vi "Dashboard Main.vi"() -> ()   [LabVIEW 2011]
uses:
  <vilib>/Rock Robotics/WPI/DriverStation/DriverStationLCD/WPI_DriverStationLCDLCDLine.ctl
  DStoPCPacketTypeDef.ctl
  <vilib>/Rock Robotics/WPI/DriverStation/WPI_DriverStationDigitalData.ctl
panel:
  out "SPEED":dbl(knob) scale=0.1..100.0
  out "8 -- Battery":sgl(graph)
  out "Analog Input":sgl[](array[slide]) scale=0.0..5.0
  in  "Viewer":enum32{"Camera Image", "Kinect Skeleton"}(tab)
  in  "Video Enable":bool=TRUE
  out "Camera Image":T1(plugin-control)
  out "Buttons 1":cluster{"1":bool, "2":bool, "3":bool}
  out "Kinect 1":cluster{"X":dbl, "Y":dbl, "Z":dbl} {"X" scale=1.0..-1.0; "Y" scale=1.0..-1.0; "Z" scale=1.0..-1.0}
  out "Buttons 2":cluster{"1":bool, "2":bool, "3":bool}
  out "Kinect 2":cluster{"X":dbl, "Y":dbl, "Z":dbl} {"X" scale=1.0..-1.0; "Y" scale=1.0..-1.0; "Z" scale=1.0..-1.0}
  out "Version":string
  out "Skeleton Picture":picture
  out "Players":i8
  out "Dashboard Datatype Warning":string="Warning: The Dashboard Datatype used by the robot project and this dashboard do not match.\nSee diagram for more details."
  out "Robot IP Address":string
  out "Image Error Message":string="Timeout in Camera Communications"
  out "Solenoid Output":bool[](array[boolean])
  out "PWM":cluster{u8, u8}[](array[slide])=[{0, 157}, {0, 157}, {0, 157}, {0, 157}, {0, 157}, {0, 157}, {0, 157}, {0, 157}, {0, 157}, {0, 169}] scale=1.0..255.0
  out "GPIO Output Enable":bool[](array[boolean])
  out "GPIO State":bool[](array[boolean])
  out "Relay":cluster{"Forward":bool[], "Reverse":bool[]}
  # "Analog #1"
  # "1"
  # "7"
  # "Communications"
  # "Solenoid #1"
  # "1"
  # "8"
  # "Digital #1"
  # "1"
  # "10"
  # "1"
  # "14"
  # "1"
  # "8"
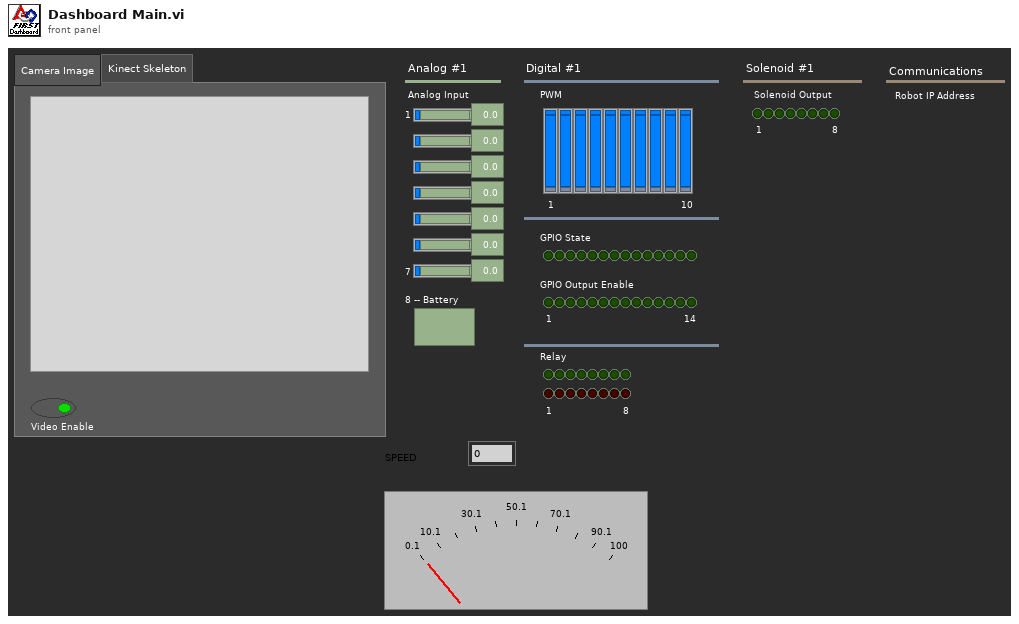
[diagram p1: front panel]
types:
  T1 = typedef "IMAQ Image.ctl" = refnum<image>
  T2 = typedef "DStoPCPacketTypeDef.ctl" = cluster{"Packet Index":u16, "Digital Inputs":u8, "Digital Out":u8, "Battery":u16, "Status":u8, "Error":u8, "Team ID":u16, "VersionMonth1":u8, "VersionMonth2":u8, "VersionDay1":u8, "VersionDay2":u8, "VersionYear1":u8, "VersionYear2":u8, "Revision1":u8, "Revision2":u8, "UnusedBuffer":u32, "UnusedBuffer 2":u16, "Reply Packet #":u16, "SPEED":dbl}
  T3 = cluster{"AnalogModule[0]":cluster{"Channel[3]":sgl}, "AnalogModule[1]":cluster{"Channel[1]":sgl}, "Cluster":T2}
  T4 = typedef "WPI_DriverStationDigitalData.ctl" = cluster{"Relay Fwd":u8, "Relay Rev":u8, "GPIO":u16, "GPIO_OE":u16, "PWM":cluster{"PWM[0]":u8, "PWM[1]":u8, "PWM[2]":u8, "PWM[3]":u8, "PWM[4]":u8, "PWM[5]":u8, "PWM[6]":u8, "PWM[7]":u8, "PWM[8]":u8, "PWM[9]":u8}}
  T5 = cluster{cluster{"AnalogModule[0]":cluster{"Channel[0]":sgl, "Channel[1]":sgl, "Channel[2]":sgl, "Channel[3]":sgl, "Channel[4]":sgl, "Channel[5]":sgl, "Channel[6]":sgl, "Channel[7]":sgl}, "AnalogModule[1]":cluster{"Channel[0]":sgl, "Channel[1]":sgl, "Channel[2]":sgl, "Channel[3]":sgl, "Channel[4]":sgl, "Channel[5]":sgl, "Channel[6]":sgl, "Channel[7]":sgl}}, cluster{"DigitalModule[0]":T4}, "Solenoid":u8, "DigitalModule[1]":T4}
  T6 = typedef "Image Type" = u32
  T7 = cluster{"Competition mode":bool, "Robot Link":bool, "Autonomous":bool, "Enabled":bool, "E-Stop":bool}
  T8 = cluster{"AnalogModule[0]":cluster{"Channel[0]":sgl, "Channel[1]":sgl, "Channel[2]":sgl, "Channel[3]":sgl, "Channel[4]":sgl, "Channel[5]":sgl, "Channel[6]":sgl, "Channel[7]":sgl}, "AnalogModule[1]":cluster{"Channel[0]":sgl, "Channel[1]":sgl, "Channel[2]":sgl, "Channel[3]":sgl, "Channel[4]":sgl, "Channel[5]":sgl, "Channel[6]":sgl, "Channel[7]":sgl}}
  T9 = cluster{"Channel[0]":sgl, "Channel[1]":sgl, "Channel[2]":sgl, "Channel[3]":sgl, "Channel[4]":sgl, "Channel[5]":sgl, "Channel[6]":sgl, "Channel[7]":sgl}[]
  T10 = cluster{"Channel[0]":sgl, "Channel[1]":sgl, "Channel[2]":sgl, "Channel[3]":sgl, "Channel[4]":sgl, "Channel[5]":sgl, "Channel[6]":sgl, "Channel[7]":sgl}
  T11 = typedef "LVRectTypeDef.ctl" = cluster{"left":i16, "top":i16, "right":i16, "bottom":i16}
  T12 = typedef "SkeletonTrackState.ctl" = enum32{"NotTracked", "PositionOnly", "Tracked"}
  T13 = cluster{"TrackingState":u8[], "Position":cluster{"x":sgl, "y":sgl, "z":sgl}, cluster{"x":sgl, "y":sgl, "z":sgl, sgl}[], "TrackState":T12}
  T14 = cluster{cluster{"ScaledToPercentRange":dbl, "ScaledToPercentRange":dbl, "ScaledToPercentRange":dbl}, cluster{bool, bool, bool}}[]
  T15 = typedef "LVBoundsTypeDef.ctl" = cluster{"Width":u32, "Height":u32}
  T16 = cluster{cluster{"ScaledToPercentRange":dbl, "ScaledToPercentRange":dbl, "ScaledToPercentRange":dbl}, cluster{bool, bool, bool}}
  T17 = cluster{"ScaledToPercentRange":dbl, "ScaledToPercentRange":dbl, "ScaledToPercentRange":dbl}
  T18 = typedef "WPI_DriverStationLCDLCDLine.ctl" = enum16{"Main - Line 1", "User - Line 2", "User - Line 3", "User - Line 4", "User - Line 5", "User - Line 6"}
  T19 = typedef "WPI_EncoderDevRef.ctl" = cluster{"DevStatus":errorcluster, "EncoderIndex":T20, "CounterIndex":T21, "DistancePerCount":dbl, "Decoding Type":T22}
  T20 = typedef "FPGA_EncoderIdx.ctl" = enum8{"Enc 0", "Enc 1", "Enc 2", "Enc 3", "Invalid"}
  T21 = typedef "FPGA_CounterCtrSystemIndex.ctl" = enum8{"Ctr 0", "Ctr 1", "Ctr 2", "Ctr 3", "Ctr 4", "Ctr 5", "Ctr 6", "Ctr 7", "Invalid"}
  T22 = typedef "WPI_EncoderType.ctl" = enum16{"1x", "2x", "4x"}
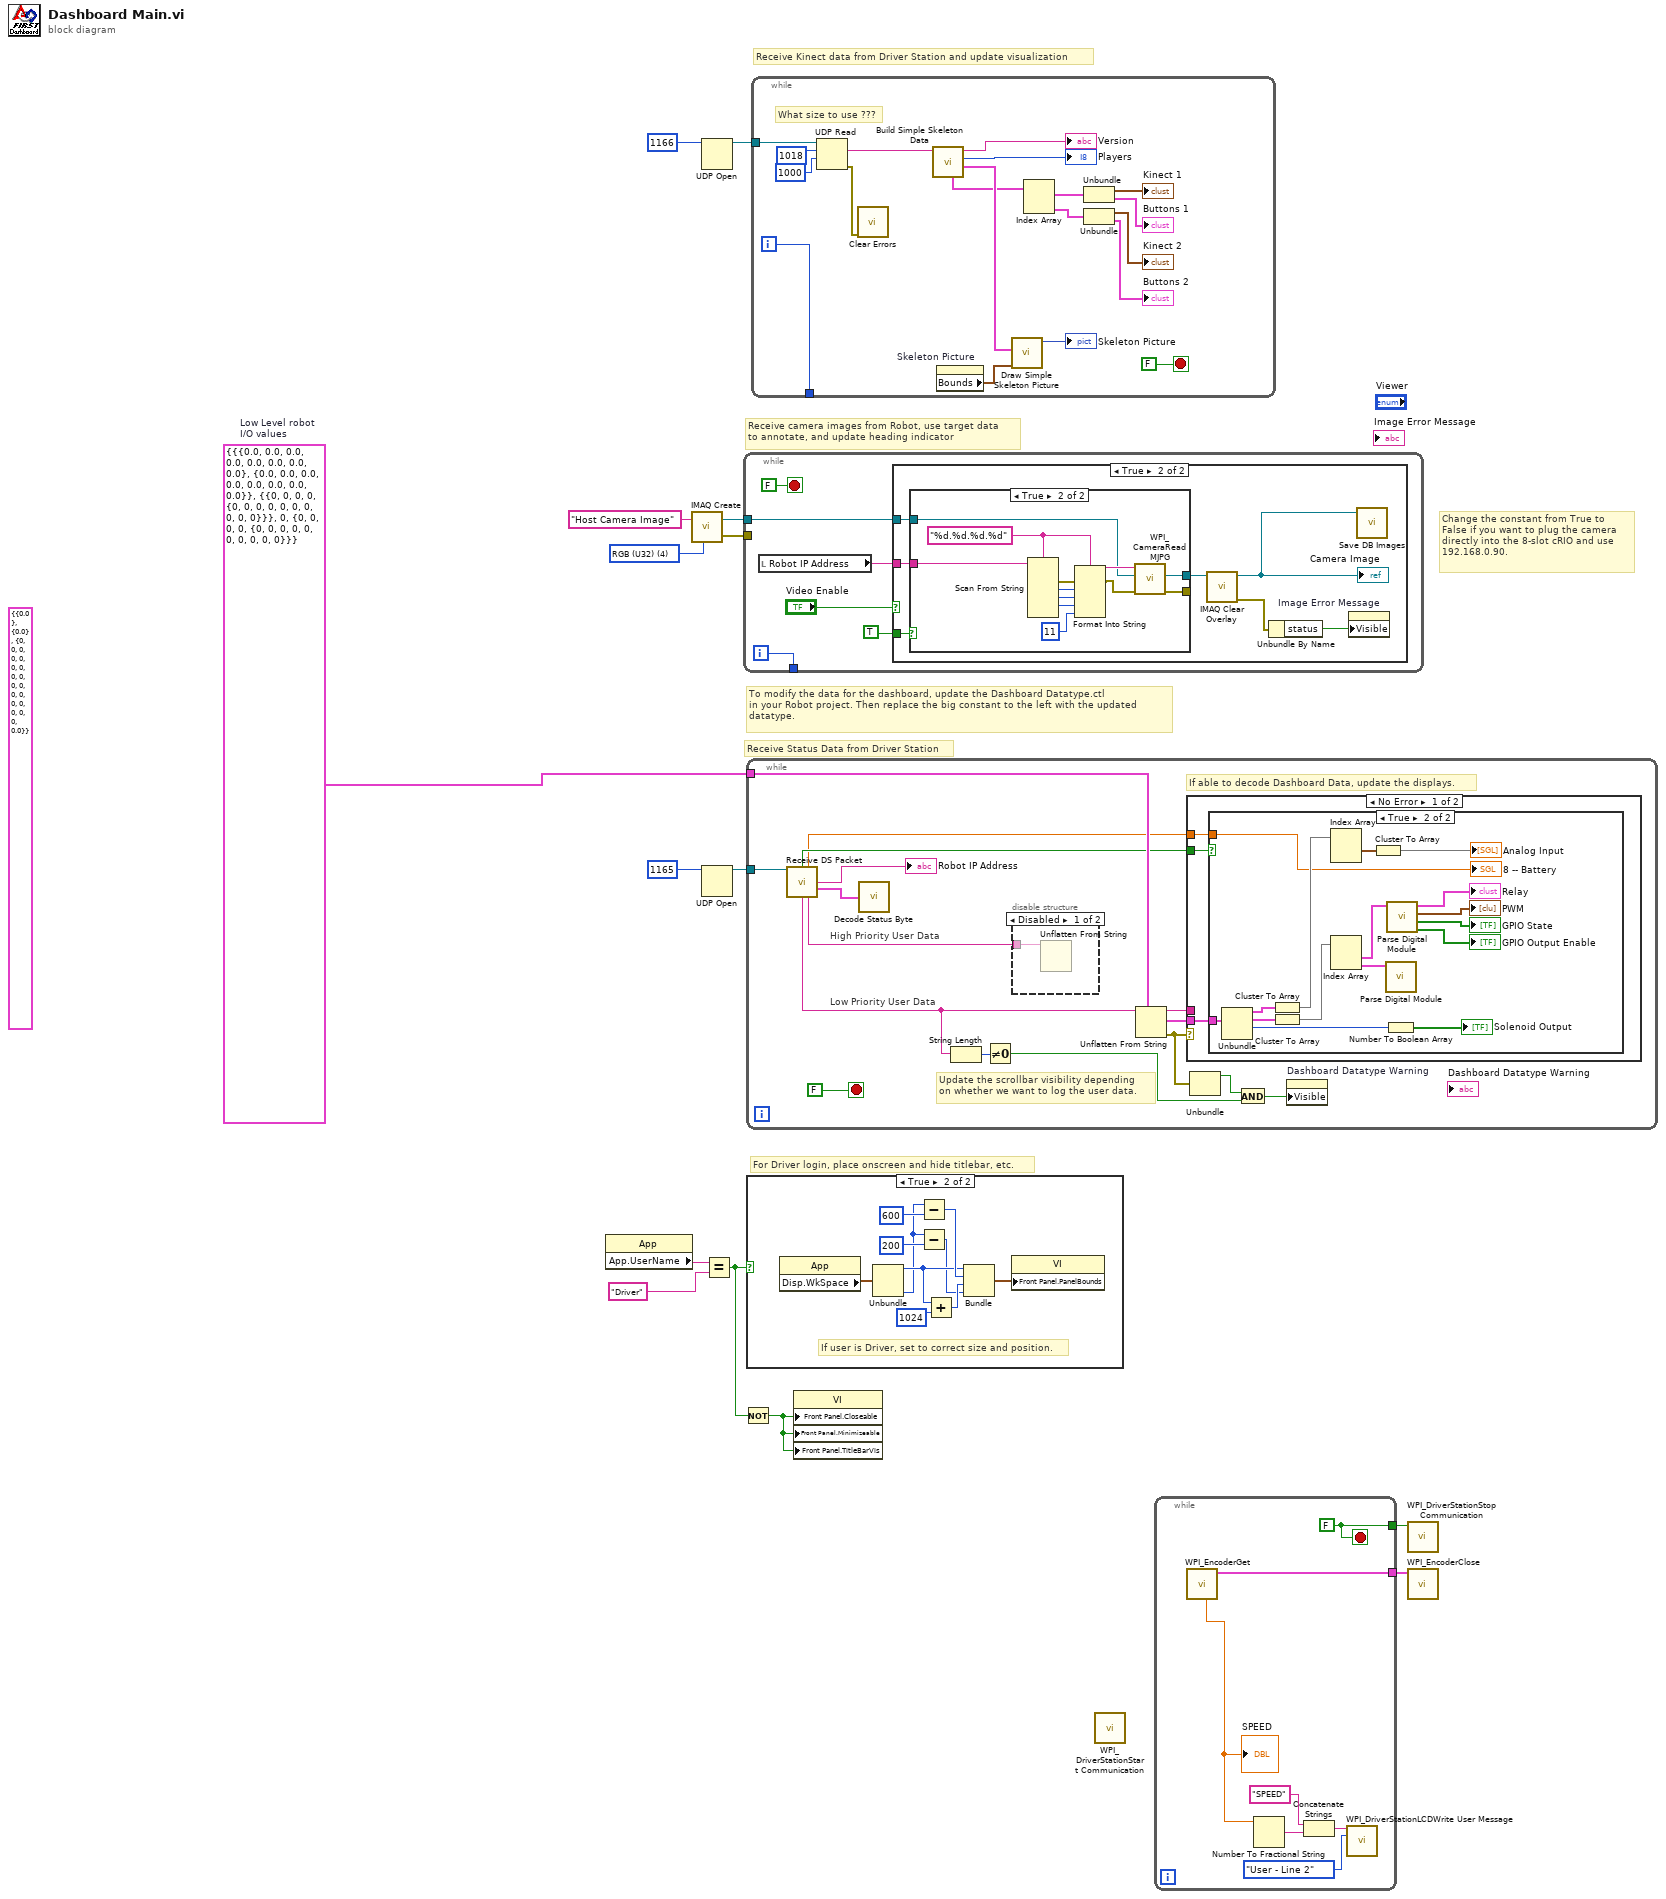
[diagram p0: block diagram]
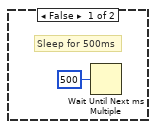
[diagram p6: hidden frame]
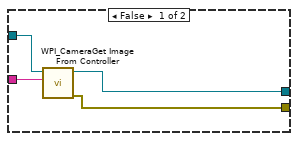
[diagram p7: hidden frame]
diagram:
  (unwired) T3 {"AnalogModule[0]"={"Channel[3]"=0.0}, "AnalogModule[1]"={"Channel[1]"=0.0}, "Cluster"={"Packet Index"=0, "Digital Inputs"=0, "Digital Out"=0, "Battery"=0, "Status"=0, "Error"=0, "Team ID"=0, "VersionMonth1"=0, "VersionMonth2"=0, "VersionDay1"=0, "VersionDay2"=0, "VersionYear1"=0, "VersionYear2"=0, "Revision1"=0, "Revision2"=0, "UnusedBuffer"=0, "UnusedBuffer 2"=0, "Reply Packet #"=0, "SPEED"=0.0}}
  w1 = T5 {{"AnalogModule[0]"={"Channel[0]"=0.0, "Channel[1]"=0.0, "Channel[2]"=0.0, "Channel[3]"=0.0, "Channel[4]"=0.0, "Channel[5]"=0.0, "Channel[6]"=0.0, "Channel[7]"=0.0}, "AnalogModule[1]"={"Channel[0]"=0.0, "Channel[1]"=0.0, "Channel[2]"=0.0, "Channel[3]"=0.0, "Channel[4]"=0.0, "Channel[5]"=0.0, "Channel[6]"=0.0, "Channel[7]"=0.0}}, {"DigitalModule[0]"={"Relay Fwd"=0, "Relay Rev"=0, "GPIO"=0, "GPIO_OE"=0, "PWM"={"PWM[0]"=0, "PWM[1]"=0, "PWM[2]"=0, "PWM[3]"=0, "PWM[4]"=0, "PWM[5]"=0, "PWM[6]"=0, "PWM[7]"=0, "PWM[8]"=0, "PWM[9]"=0}}}, "Solenoid"=0, "DigitalModule[1]"={"Relay Fwd"=0, "Relay Rev"=0, "GPIO"=0, "GPIO_OE"=0, "PWM"={"PWM[0]"=0, "PWM[1]"=0, "PWM[2]"=0, "PWM[3]"=0, "PWM[4]"=0, "PWM[5]"=0, "PWM[6]"=0, "PWM[7]"=0, "PWM[8]"=0, "PWM[9]"=0}}}  # Low Level robot I/O values
  w13 = T6 4 items=["Grayscale (U8)", "Grayscale (I16)", "Grayscale (SGL)", "Complex (CSG)", "RGB (U32)", "HSL (U32)", "RGB (U64)"] ("Image Type")
  # "Change the constant from True to\nFalse if you want to plug the camera\ndirectly into the 8-slot cRIO and use\n192.168.0.90."
  # "Receive Kinect data from Driver Station and update visualization"
  # "For Driver login, place onscreen and hide titlebar, etc."
  # "To modify the data for the dashboard, update the Dashboard Datatype.ctl\nin your Robot project. Then replace the big constant to the left with the updated\ndatatype."
  # "Receive Status Data from Driver Station"
  # "Receive camera images from Robot, use target data\nto annotate, and update heading indicator"
  n1 = property class="App"() -> ("App.UserName"=w8:string)  [unwired: 2 in, 2 out]
  n2 = call "IMAQ Create"("Image Name"="Host Camera Image", "Image Type"=w13) -> ("New Image"=w11:T1, "error out"=w10:errorcluster)  [unwired: 2 in, 1 out]
  n3 = UDP Open(11:u16 1166 ("port")) -> (port=w4:refnum<k16>)  [unwired: 2 in, 4 out]
  n4 = UDP Open(11:u16 1165 ("port")) -> (port=w14:refnum<k16>)  [unwired: 2 in, 4 out]
  n5 = Equal?(x=w8, y="Driver") -> (x = y?=w7:bool)
  n6 = Not(x=w7) -> (.not. x?=w6:bool)
  n7 = while {
    tunnel: w11 -> [w19]
    tunnel: w10 -> [_]
    tunnel: [w16] -> _
    i -> [w16]
    stop <- FALSE stop-if-true
    n8 = local read "Robot IP Address"() -> (w20:string)
    n9 = case shown="True" "Video Enable" {
      tunnel: w20 -> [_ w29]
      tunnel: w19 -> [_ w28]
      tunnel: TRUE -> [_ w23]
      frame False {
        # "Sleep for 500ms"
        n10 = Wait Until Next ms Multiple(millisecond multiple=u32 500) -> ()  [unwired: 1 out]
      }
      frame True {
        n11 = case shown="True" w23 {
          tunnel: w28 -> [w32 w39]
          tunnel: [w30 w37] -> _
          tunnel: [w31 w38] -> w25
          tunnel: w29 -> [w33 w42]
          frame False {
            n12 = call <vilib>:"WPI_CameraGet Image From Controller.vi"("Controller Address"=w33, "Image"=w32) -> ("error out"=w30:errorcluster, "Image Out"=w31:T1)  [unwired: 2 in, 6 out]
          }
          frame True {
            w34 = "%d.%d.%d.%d" ("format string")
            n13 = Scan From String(format string=w34, input string=w42) -> (error out=w41:errorcluster, output 1=w43:i32, output 2=w44:i32, output 3=w45:i32)  [unwired: 2 in, 7 out]
            n14 = Format Into String(format string=w34, error in=w41, w43, w44, w45, 11 ("IP Suffix:")) -> (resulting string=w40:string, error out=w36:errorcluster)  [unwired: 1 in]
            n15 = call <vilib>:"WPI_CameraRead MJPG.vi"("error in"=w36, "Image"=w39, "address"=w40) -> ("error out"=w37:errorcluster, "Image Out"=w38:T1)  [unwired: 7 in]
          }
        }
        n16 = call "IMAQ Clear Overlay"("Image"=w25) -> ("error out"=w26:errorcluster, "Image Out"=w24:T1)  [unwired: 2 in, 7 out]
        "Camera Image" <- w24
        n17 = Unbundle By Name(w26) -> ("status"=w27:bool)
        n18 = property on="Image Error Message" class="Str"("Visible"=w27) -> ()  [unwired: 2 in, 2 out]
        n19 = call "Save DB Images.vi"("Image"=w24) -> ()  [unwired: 2 in, 1 out]
      }
    }
  }
  n20 = while {
    tunnel: w14 -> [w59]
    tunnel: w1 -> [w58]
    stop <- FALSE stop-if-true
    # "High Priority User Data"
    # "Low Priority User Data"
    # "Update the scrollbar visibility depending\non whether we want to log the user data."
    # "If able to decode Dashboard Data, update the displays."
    n21 = call "Receive DS Packet.vi"("Recv Socket"=w59) -> ("New Dashboard Data"=w55:bool, "Battery"=w46:sgl, "Robot IP Address"=→"Robot IP Address":string, "Status"=w60:T7, "Low Priority User Data"=w48:string, "High Priority User Data"=w47:string)  [unwired: 1 in, 8 out]
    n22 = call "Decode Status Byte.vi"("Status Byte"=w60) -> ()  [unwired: 2 out]
    n23 = String Length(string=w48) -> (length=w50:i32)
    n24 = Not Equal To 0?(x=w50) -> (x != 0?=w53:bool)
    n25 = disable-structure shown="Disabled" {
      disable-tunnel: w47 -> [w62 _]
      frame Disabled {
        n26 = Unflatten From String(binary string=w62) -> ()  [unwired: 2 in, 5 out]
      }
      frame Enabled {
      }
    }
    n27 = Unflatten From String(type=w58, binary string=w48) -> (rest of the binary string=w51:string, value=w57:T5, error out=w56:errorcluster)  [unwired: 1 in, 2 out]
    n28 = case shown="No Error" w56 {
      tunnel: w57 -> [w65 _]
      tunnel: w55 -> [w64 _]
      tunnel: w51 -> [_ _]
      tunnel: w46 -> [w63 _]
      frame No Error {
        n29 = case shown="True" w64 {
          tunnel: w65 -> [_ w72]
          tunnel: w63 -> [_ w66]
          frame False {
            # "Don't update if the robot hasn't sent new data"
          }
          frame True {
            n30 = Unbundle(w72) -> (w69:T8, w70:cluster{"DigitalModule[0]":T4}, "Solenoid"=w71:u8)  [unwired: 1 out]
            n31 = Cluster To Array(cluster=w69) -> (array=w80:T9)
            n32 = Cluster To Array(cluster=w70) -> (array=w79:T4[])
            n33 = Index Array(array=w80) -> (element #1=w67:T10)  [unwired: 2 in, 1 out]
            n34 = Index Array(array=w79) -> (element #1=w78:T4, element #2=w73:T4)  [unwired: 2 in]
            n35 = Cluster To Array(cluster=w67) -> (array=→"Analog Input":sgl[])
            n36 = call "Parse Digital Module.vi"("DigitalModule"=w73) -> ()  [unwired: 11 out]
            n37 = Number To Boolean Array(number=w71) -> (Boolean array=→"Solenoid Output":bool[])
            n38 = call "Parse Digital Module.vi"("DigitalModule"=w78) -> ("GPIO Output Enable"=→"GPIO Output Enable":bool[], "GPIO State"=→"GPIO State":bool[], "PWM"=→"PWM":cluster{u8, u8}[], "Relay"=→"Relay":cluster{"Forward":bool[], "Reverse":bool[]})  [unwired: 7 out]
            "8 -- Battery" <- w66
          }
        }
      }
      frame Error {
        # "Your datatypes don't match. The Dashboard Datatype.ctl in your Robot project\nand the big constant to the left of the loop need to match."
      }
    }
    n39 = Unbundle(w56) -> ("status"=w52:bool)  [unwired: 2 out]
    n40 = And(x=w52, y=w53) -> (x .and. y?=w54:bool)
    n41 = property on="Dashboard Datatype Warning" class="Str"("Visible"=w54) -> ()  [unwired: 2 in, 2 out]
  }
  n42 = case shown="True" w7 {
    frame False {
    }
    frame True {
      # "If user is Driver, set to correct size and position."
      n43 = property class="App"() -> ("Disp.WkSpace"=w91:T11)  [unwired: 2 in, 2 out]
      n44 = Unbundle(w91) -> ("left"=w86:i16, "bottom"=w82:i16)  [unwired: 2 out]
      n45 = Subtract(x=w82, y=600) -> (x-y=w88:i32)
      n46 = Subtract(x=w82, y=200) -> (x-y=w83:i32)
      n47 = Add(x=w86, y=1024) -> (x+y=w87:i32)
      n48 = Bundle("left"=w86, w88, w87, w83) -> (w90:cluster{"left":i16, i32, i32, i32})  [unwired: 1 out]
      n49 = property class="VI"("Front Panel.PanelBounds"=w90) -> ()  [unwired: 2 in, 2 out]
    }
  }
  n50 = while {
    tunnel: w4 -> [w108]
    tunnel: [w92] -> _
    i -> [w92]
    stop <- FALSE stop-if-true
    # "What size to use ???"
    n51 = UDP Read(connection ID=w108, max size (548)=1018 ("bytes to read"), timeout ms (25000)=1000) -> (data out=w102:string, error out=w100:errorcluster)  [unwired: 1 in, 3 out]
    n52 = call <vilib>:"Clear Errors.vi"("error in (no error)"=w100) -> ()  [unwired: 6 in, 1 out]
    n53 = call "Build Simple Skeleton Data.vi"("data out"=w102) -> ("Skeleton Data"=w103:T13, "NumPlayers"=→"Players":i8, "Version String"=→"Version":string, "Simple Joystick Info"=w99:T14)  [unwired: 6 in, 1 out]
    n54 = property on="Skeleton Picture" class="Pict"() -> ("Bounds"=w104:T15)  [unwired: 2 in, 2 out]
    n55 = call "Draw Simple Skeleton Picture.vi"("Bounds"=w104, "Simple Skeleton"=w103) -> ("new picture out"=→"Skeleton Picture":picture)  [unwired: 9 in]
    n56 = Index Array(array=w99) -> (element #1=w98:T16, element #2=w97:T16)  [unwired: 2 in]
    n57 = Unbundle(w98) -> (→"Kinect 1":T17, →"Buttons 1":cluster{bool, bool, bool})
    n58 = Unbundle(w97) -> (→"Kinect 2":T17, →"Buttons 2":cluster{bool, bool, bool})
  }
  n59 = property class="VI"("Front Panel.Closeable"=w6, "Front Panel.Minimizeable"=w6, "Front Panel.TitleBarVis"=w6) -> ()  [unwired: 2 in, 2 out]
  n60 = call <vilib>:"WPI_DriverStationStart Communication.vi"() -> ()  [unwired: 12 in]
  n61 = while {
    tunnel: [w117] -> w3
    tunnel: [w111] -> w2
    stop <- w111 stop-if-true
    w111 = FALSE
    n62 = call <vilib>:"WPI_EncoderGet.vi"() -> ("EncoderDevRef"=w117:T19, "Rate"=w113:dbl)  [unwired: 6 in, 4 out]
    "SPEED" <- w113
    n63 = Number To Fractional String(number=w113) -> (F-format string=w115:string)  [unwired: 3 in]
    n64 = Concatenate Strings("SPEED" ("string"), w115) -> (w114:string)
    n65 = call <vilib>:"WPI_DriverStationLCDWrite User Message.vi"("line text"=w114, "line"=WPI_DriverStationLCDLCDLine."User - Line 2") -> ()  [unwired: 13 in, 1 out]
  }
  n66 = call <vilib>:"WPI_DriverStationStop Communication.vi"("StopCommunication"=w2) -> ()  [unwired: 10 in, 1 out]
  n67 = call <vilib>:"WPI_EncoderClose.vi"("EncoderDevRef"=w3) -> ()  [unwired: 10 in, 1 out]
